vi "Convert Unit.vi"(8 "error in (no error)":errorcluster, 9 "value":dbl, 10 "unit to (air)":T1=1 items=["cReturnWavelengthVac", "cReturnWavelengthAir", "cReturnFrequency", "cReturnWavenumber", "cReturnPhotonEnergy"], 11 "unit from (vac)":T1 items=["cReturnWavelengthVac", "cReturnWavelengthAir", "cReturnFrequency", "cReturnWavenumber", "cReturnPhotonEnergy"]) -> (0 "error out":errorcluster, 1 "value out":dbl)   [LabVIEW 2009, in "HighFinesse WS5.lvlib"]
doc: "Converts a given wavelength (or other value) from one unit to another, using the conversion factors built into the wavelength meter program."
uses:
  HighFinesse WS5.lvlib
  Variable Typedefs.llb/Unit.ctl
  Program Files/HighFinesse/Wavelength Meter WS5 399/Com-Test/wlmData.dll
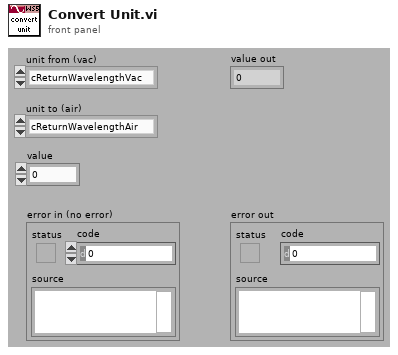
[diagram p1: front panel]
types:
  T1 = typedef "HighFinesse WS5.lvlib/Unit.ctl" = i16
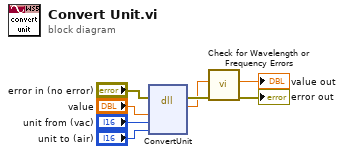
[diagram p0: block diagram]
diagram:
  n1 = dll-call lib="C:/Program Files/HighFinesse/Wavelength Meter WS5 399/Com-Test/wlmData.dll" fn="ConvertUnit"(error in="error in (no error)", "Val"="value", "uFrom"="unit from (vac)", "uTo"="unit to (air)") -> (error out=w7:errorcluster, "return type"=w6:dbl)  [unwired: 3 in, 3 out]
  n2 = call "Check for Wavelength or Frequency Errors.vi"("error in (no error)"=w7, "return code"=w6) -> ("error out"=→"error out":errorcluster, "return code out"=→"value out":dbl)  [unwired: 8 out]
